vi "ESP32_Waveform_Arduino-new.vi"(0 "headMove":dbl[](array[numeric]), 5 "beakMove":dbl[](array[numeric]), 7 "Endwert Motor1":dbl, 9 "Endwert Motor2":dbl, 11 "Sampling Rate Hz":i32, 12 "VISA resource name in":refnum<visa-resource-name>, 13 "error in":errorcluster) -> (10 "VISA resource name out":refnum<visa-resource-name>, 15 "error out":errorcluster)   [LabVIEW 2014]
panel:
  out "x*y":dbl
  out "String":string
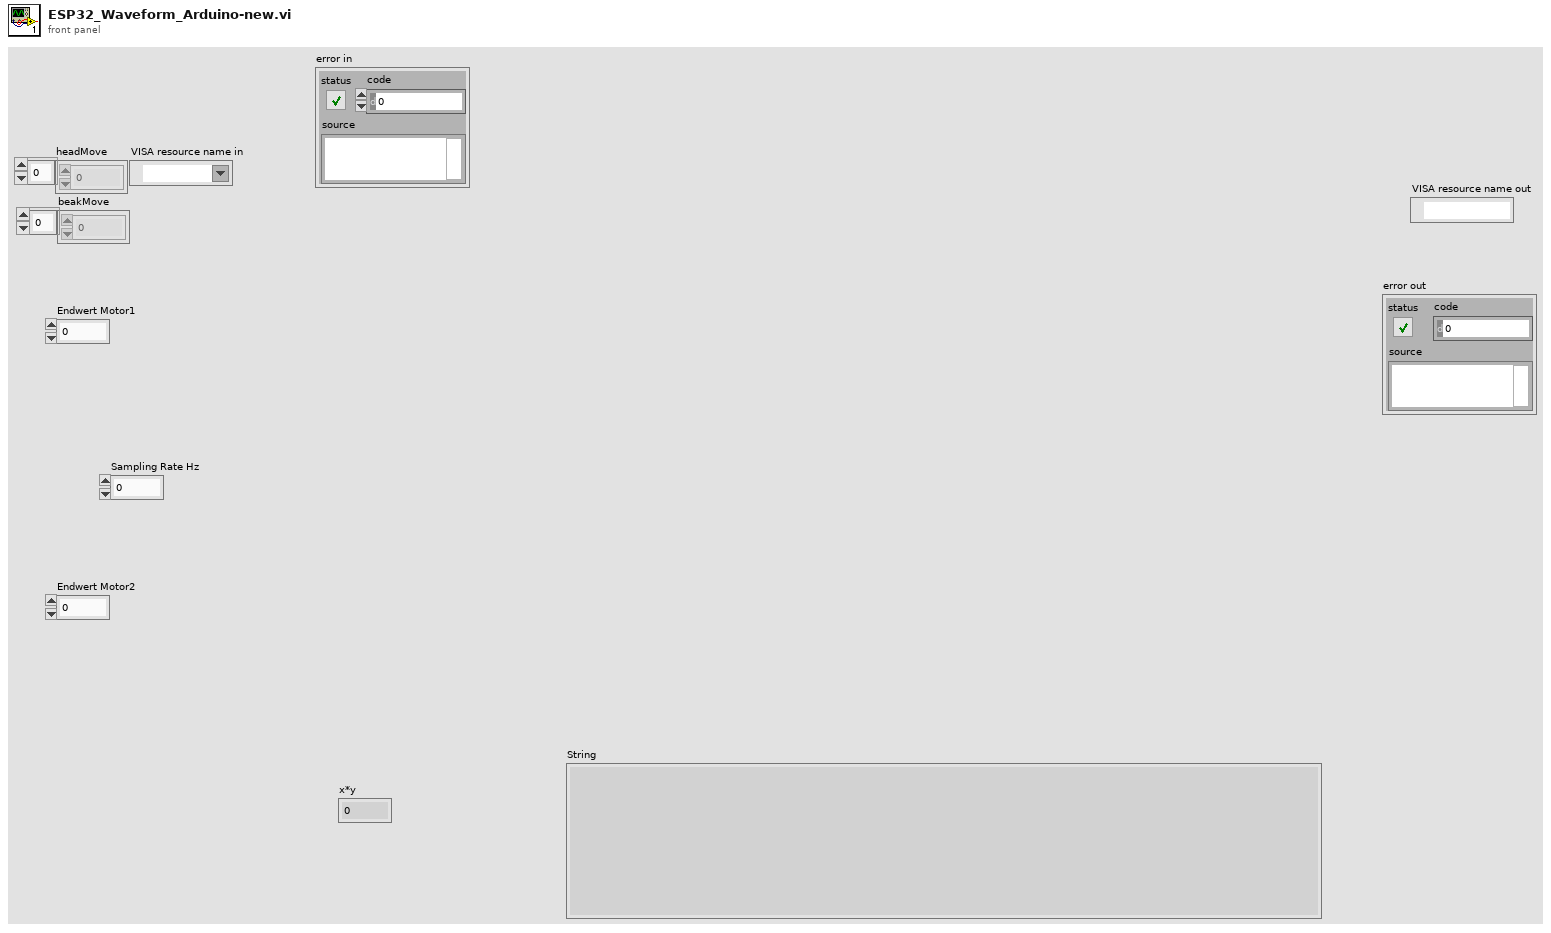
[diagram p1: front panel]
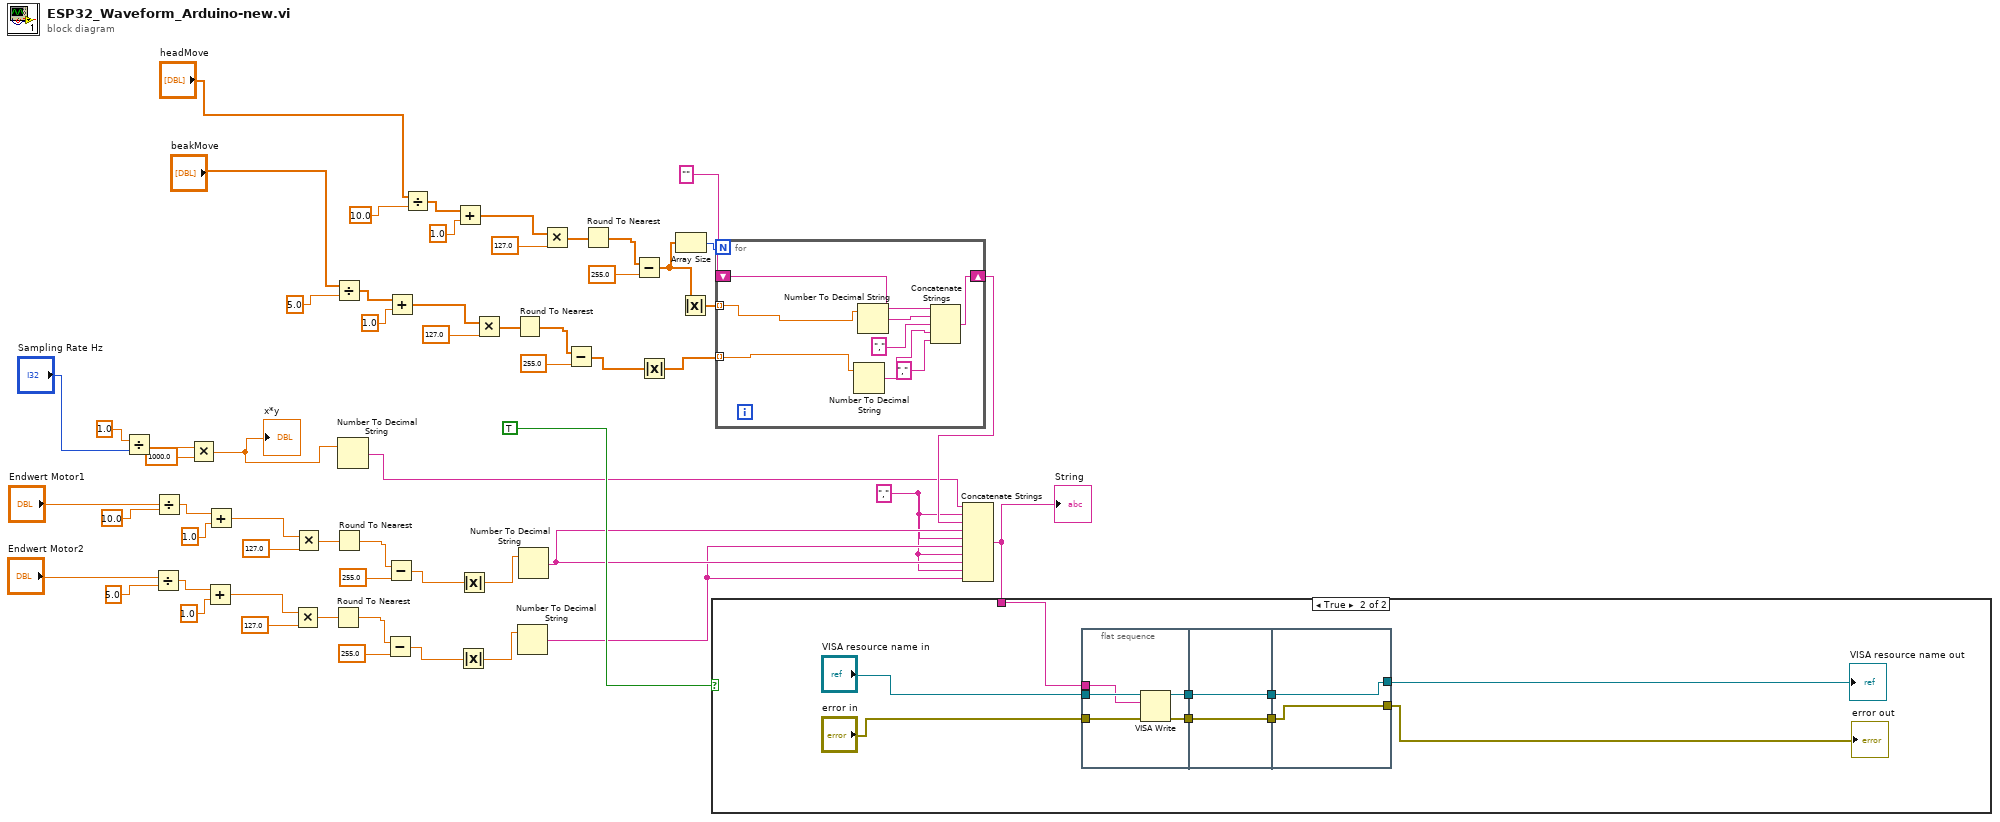
[diagram p0: block diagram]
diagram:
  w6 = ","
  n1 = Divide(x=1.0, y="Sampling Rate Hz") -> (x/y=w8:dbl)
  n2 = Divide(x="Endwert Motor2", y=5.0 ("x")) -> (x/y=w23:dbl)
  n3 = Divide(x="Endwert Motor1", y=10.0 ("x")) -> (x/y=w34:dbl)
  n4 = Multiply(x=w8, y=1000.0) -> (x*y=w5:dbl)
  "x*y" <- w5
  n5 = Add(x=w23, y=1.0 ("x")) -> (x+y=w21:dbl)
  n6 = Add(x=w34, y=1.0 ("x")) -> (x+y=w32:dbl)
  n7 = Multiply(x=w21, y=127.0 ("x")) -> (x*y=w19:dbl)
  n8 = Multiply(x=w32, y=127.0 ("x")) -> (x*y=w30:dbl)
  n9 = Round To Nearest(number=w19) -> (nearest integer value=w18:dbl)
  n10 = Divide(x="beakMove", y=5.0 ("x")) -> (x/y=w44:dbl[])
  n11 = Round To Nearest(number=w30) -> (nearest integer value=w29:dbl)
  n12 = Number To Decimal String(number=w5) -> (decimal integer string=w4:string)  [unwired: 1 in]
  n13 = Subtract(x=w18, y=255.0 ("x")) -> (x-y=w16:dbl)
  n14 = Subtract(x=w29, y=255.0 ("x")) -> (x-y=w27:dbl)
  n15 = Add(x=w44, y=1.0 ("x")) -> (x+y=w42:dbl[])
  n16 = Divide(x="headMove", y=10.0 ("x")) -> (x/y=w56:dbl[])
  n17 = Add(x=w56, y=1.0 ("x")) -> (x+y=w54:dbl[])
  n18 = Absolute Value(x=w16) -> (abs(x)=w14:dbl)
  n19 = Absolute Value(x=w27) -> (abs(x)=w25:dbl)
  n20 = Multiply(x=w42, y=127.0 ("x")) -> (x*y=w40:dbl[])
  n21 = Round To Nearest(number=w40) -> (nearest integer value=w39:dbl[])
  n22 = Number To Decimal String(number=w14) -> (decimal integer string=w10:string)  [unwired: 1 in]
  n23 = Number To Decimal String(number=w25) -> (decimal integer string=w11:string)  [unwired: 1 in]
  n24 = Multiply(x=w54, y=127.0 ("x")) -> (x*y=w52:dbl[])
  n25 = Subtract(x=w39, y=255.0 ("x")) -> (x-y=w37:dbl[])
  n26 = Round To Nearest(number=w52) -> (nearest integer value=w51:dbl[])
  n27 = Subtract(x=w51, y=255.0 ("x")) -> (x-y=w48:dbl[])
  n28 = Absolute Value(x=w37) -> (abs(x)=w36:dbl[])
  n29 = Array Size(array=w48) -> (size(s)=w49:i32)
  n30 = Absolute Value(x=w48) -> (abs(x)=w47:dbl[])
  n31 = for {
    N: w49 -> [_]
    tunnel: w47 -> [w60] mode=indexing
    shift-right: [w65] -> w13
    shift-left: "" -> [w66]
    tunnel: w36 -> [w59] mode=indexing
    n32 = Number To Decimal String(number=w59) -> (decimal integer string=w62:string)  [unwired: 1 in]
    n33 = Number To Decimal String(number=w60) -> (decimal integer string=w64:string)  [unwired: 1 in]
    n34 = Concatenate Strings(w66, w64, ",", w62, ",") -> (w65:string)
  }
  n35 = Concatenate Strings(w4, w6, w13, w11, w6, w10, w6, w11, w6, w10) -> (w12:string)
  "String" <- w12
  n36 = case shown="True" TRUE {
    tunnel: w12 -> [_ w75]
    frame False {
    }
    frame True {
      n37 = flat-sequence {
        tunnel: "VISA resource name in" -> [w80]
        tunnel: "error in" -> [w77]
        tunnel: w75 -> [w76]
        tunnel: [w79] -> w74
        tunnel: [w78] -> w73
        tunnel: w74 -> [w82]
        tunnel: w73 -> [w81]
        tunnel: [w82] -> w72
        tunnel: [w81] -> w71
        tunnel: w72 -> [w84]
        tunnel: w71 -> [w83]
        tunnel: [w83] -> w70
        tunnel: [w84] -> w69
        frame #0 {
          n38 = VISA Write(VISA resource name=w80, write buffer=w76, error in (no error)=w77) -> (VISA resource name out=w79:refnum<visa-resource-name>, error out=w78:errorcluster)  [unwired: 1 out]
        }
        frame #1 {
        }
        frame #2 {
        }
      }
      "VISA resource name out" <- w69
      "error out" <- w70
    }
  }
